vi "EMI_project_v3.vi"() -> ()   [LabVIEW 2020]
uses:
  <vilib>/Instr/_visa.llb/VISA Flush IO Buffer Mask.ctl
  <vilib>/Instr/_visa.llb/VISA Configure Serial Port (Instr).vi
panel:
  out "Fader 02 level":dbl
  out "Fader 01 level":dbl
  out "Gain Knob 02 level":dbl
  out "Gain knob 01 level":dbl
  out "manual mode led":bool
  out "Sound Balance Mode":bool
  in  "Gain Knob 02":dbl(knob) scale=0.0..270.0
  in  "Gain Knob 01":dbl(knob) scale=0.0..270.0
  in  "Fader 02 Slider":dbl(slide) scale=0.0..10.0
  in  "Fader 01 Slider":dbl(slide) scale=0.0..10.0
  out "Fader 02 Max":dbl
  out "Fader 01 Max":dbl
  in  "Calibrate":bool
  in  "stop":bool
  in  "VISA Resource":refnum<visa-resource-name>
  in  "?":bool
  in  "Gain 02":bool
  in  "?":bool
  in  "Gain 01":bool
  in  "?":bool
  in  "Fader 02":bool
  in  "?":bool
  in  "Fader 01":bool
  # "Automation System For Analog Audio Mixers"
  # "Calibration \nMode"
  # "Manual Mode"
  # "Sound Balance Mode"
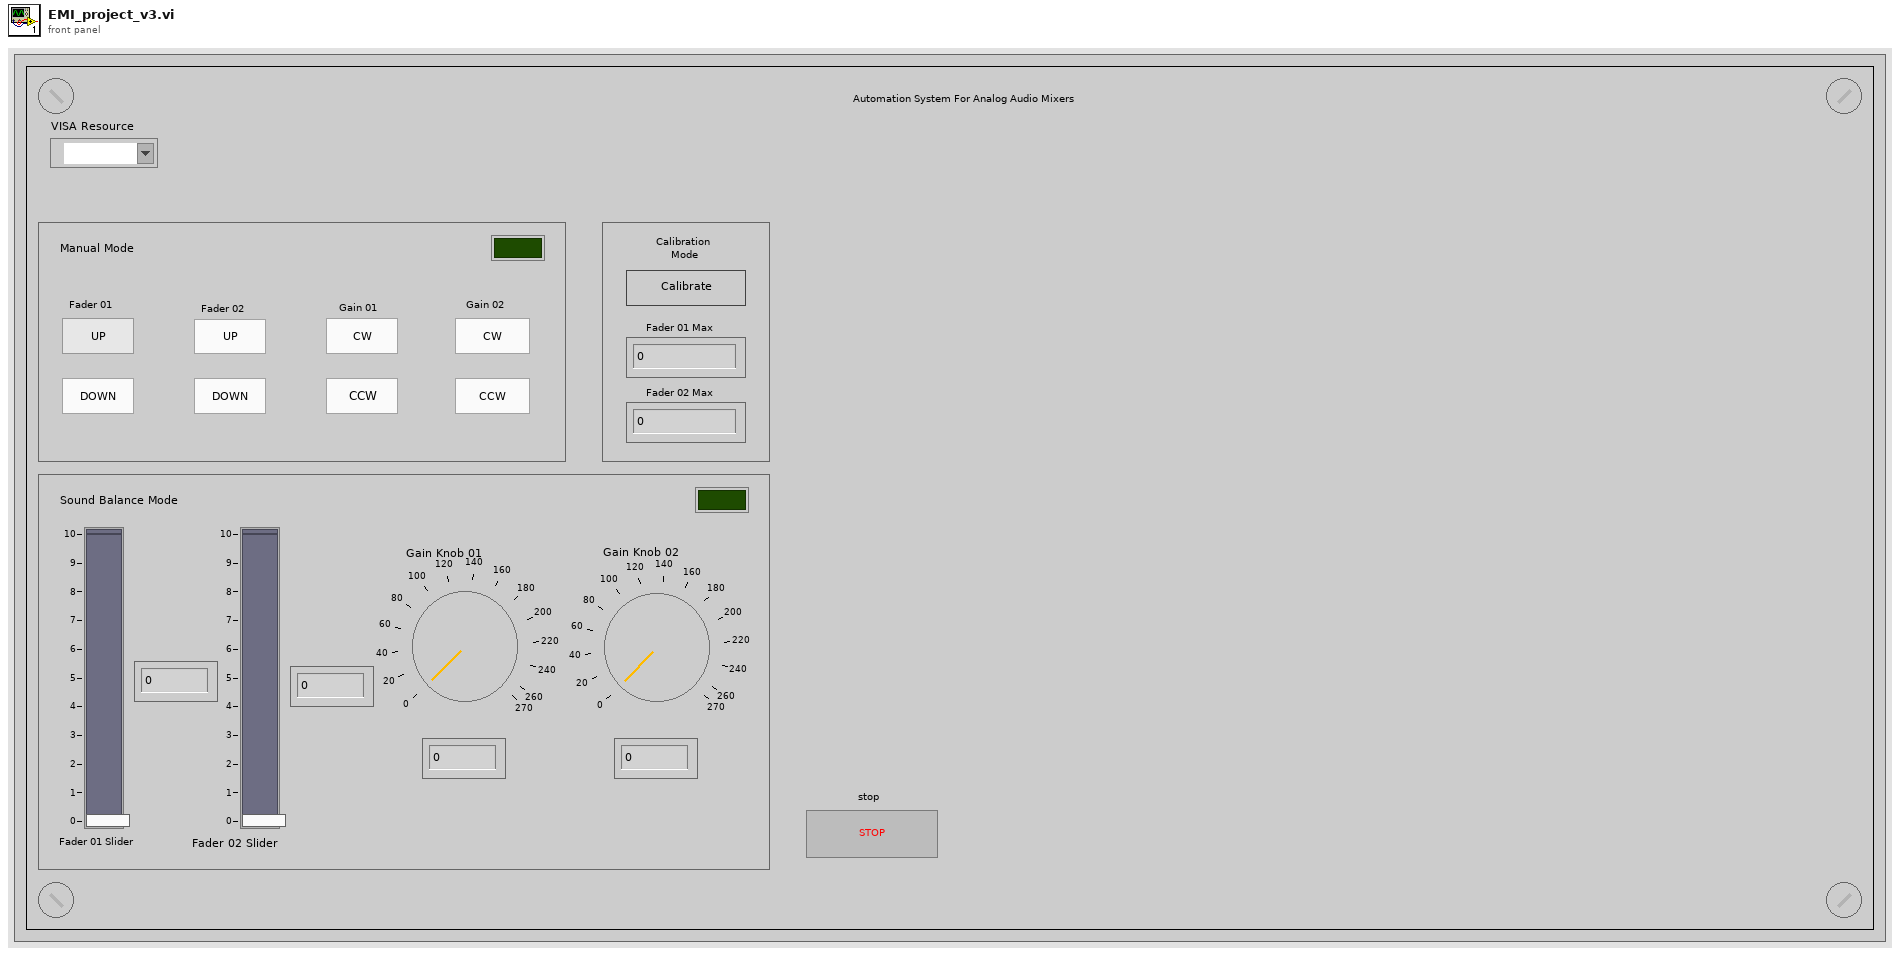
[diagram p1: front panel]
types:
  T1 = typedef "VISA Flush IO Buffer Mask.ctl" = u16
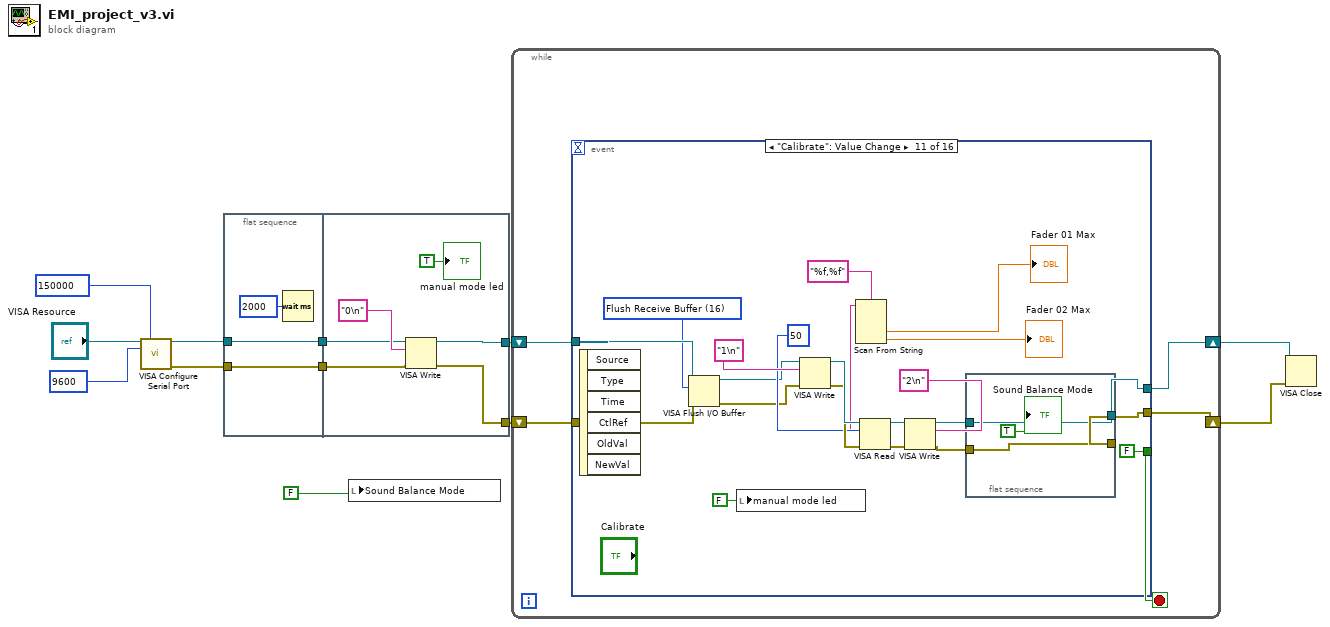
[diagram p0: block diagram]
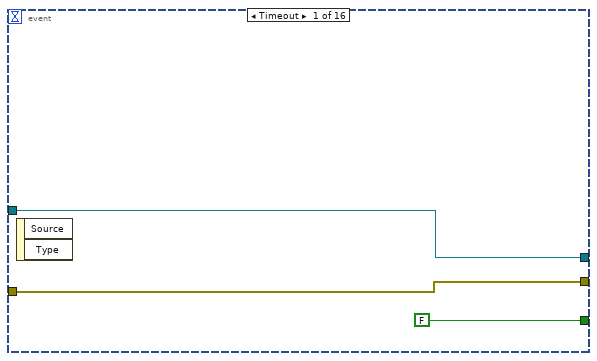
[diagram p2: hidden frame]
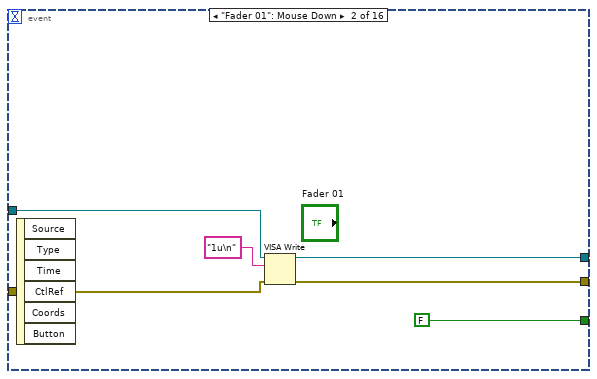
[diagram p3: hidden frame]
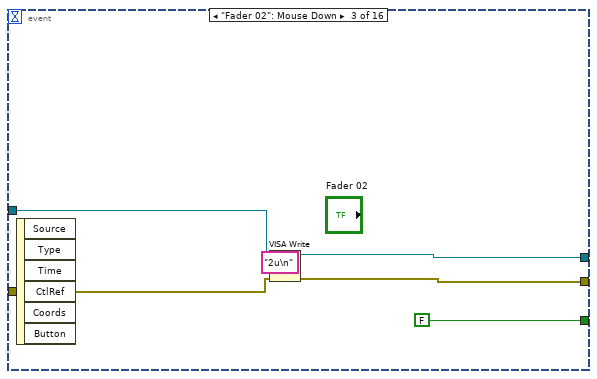
[diagram p4: hidden frame]
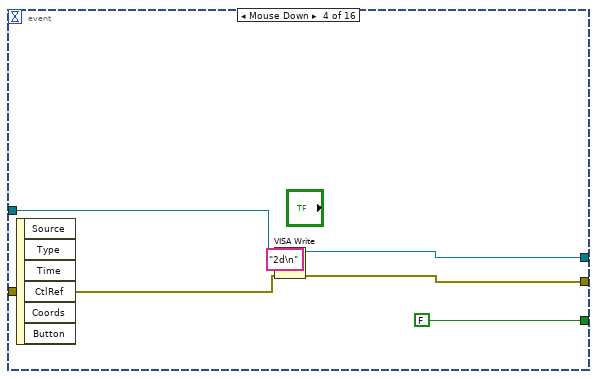
[diagram p5: hidden frame]
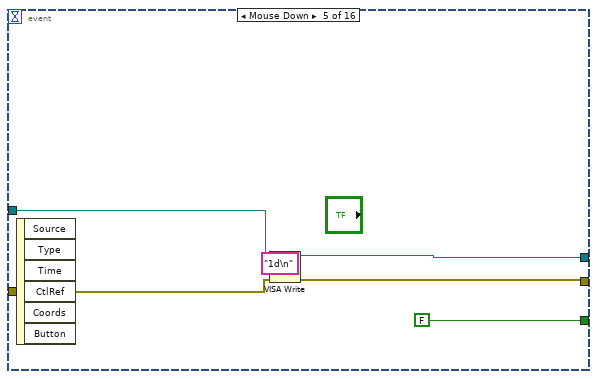
[diagram p6: hidden frame]
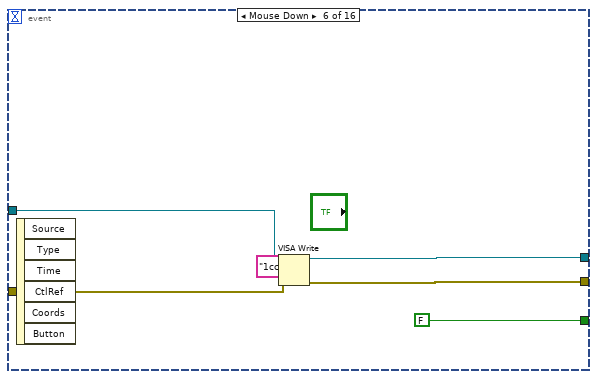
[diagram p7: hidden frame]
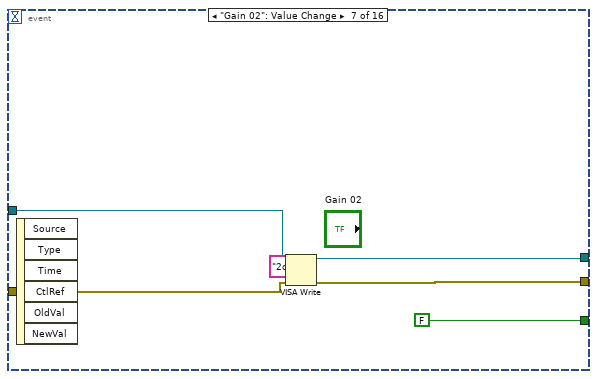
[diagram p8: hidden frame]
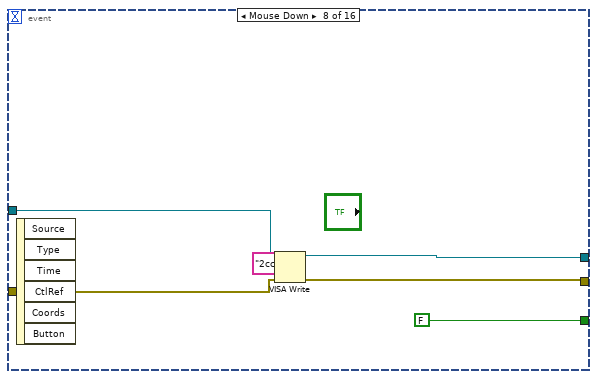
[diagram p9: hidden frame]
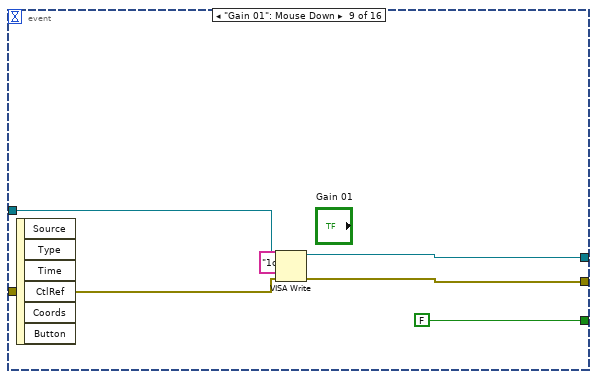
[diagram p10: hidden frame]
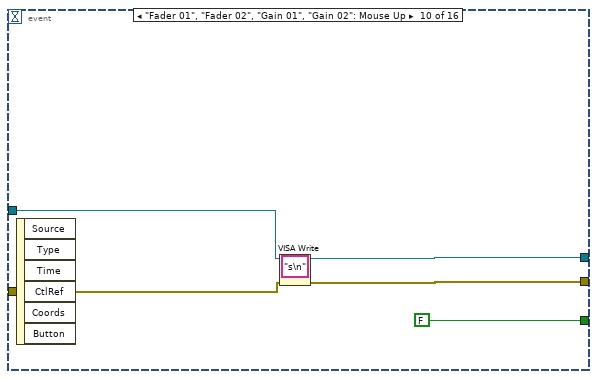
[diagram p11: hidden frame]
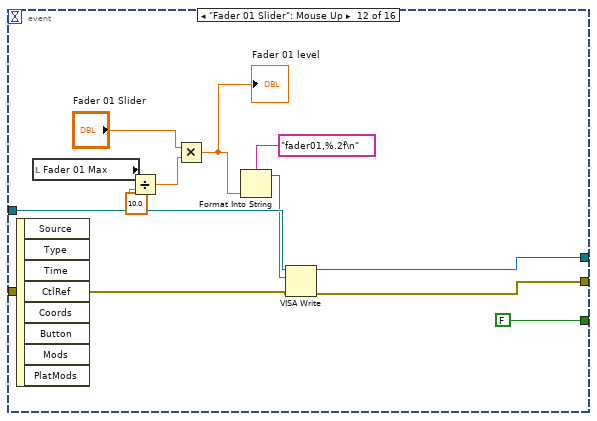
[diagram p12: hidden frame]
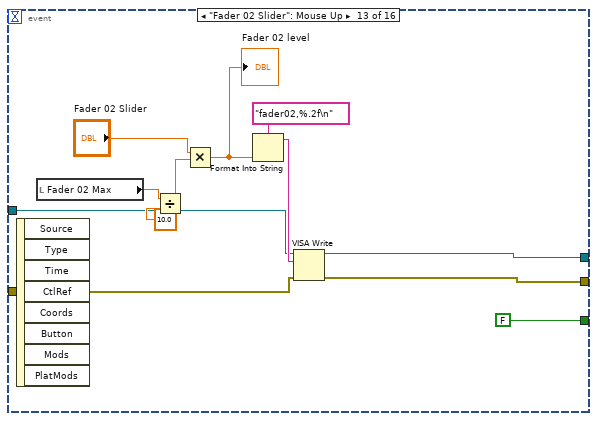
[diagram p13: hidden frame]
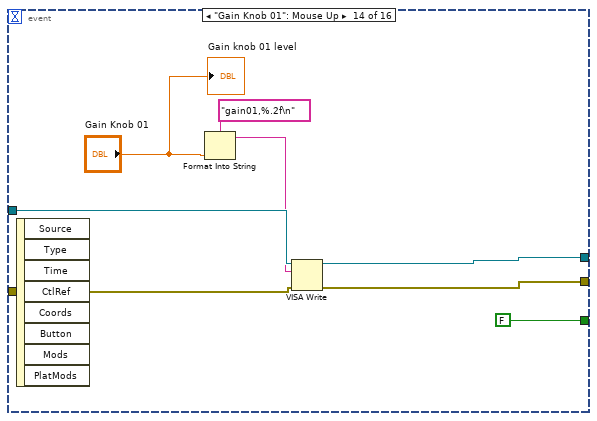
[diagram p14: hidden frame]
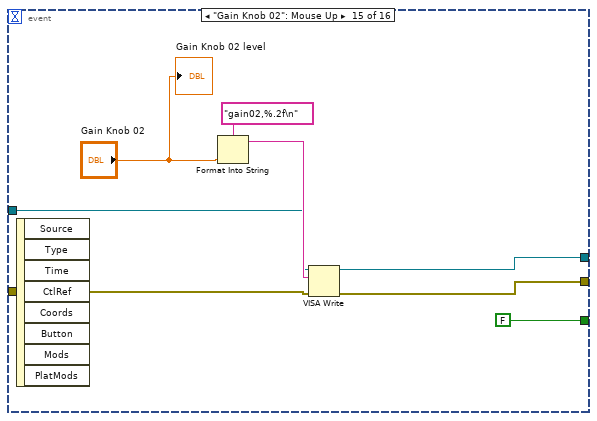
[diagram p15: hidden frame]
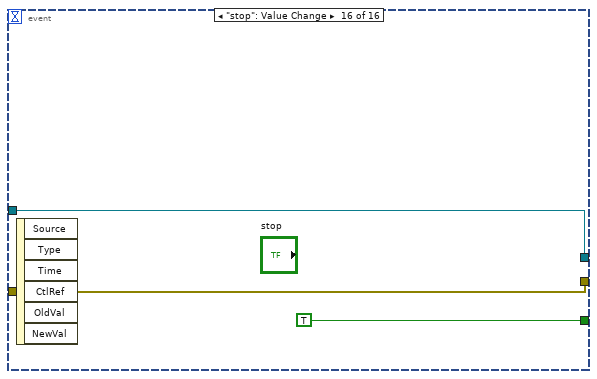
[diagram p16: hidden frame]
diagram:
  n1 = call-poly "VISA Configure Serial Port"("VISA resource name"="VISA Resource", "timeout (10sec)"=u32 150000, "baud rate (9600)"=u32 9600) -> ("VISA resource name out"=w6:refnum<visa-resource-name>, "error out"=w5:errorcluster)  [unwired: 11 in]
  n2 = flat-sequence {
    tunnel: w5 -> [w14]
    tunnel: w6 -> [w15]
    tunnel: [w15] -> w4
    tunnel: [w14] -> w3
    tunnel: [w20] -> w10
    tunnel: [w19] -> w9
    tunnel: w4 -> [w18]
    tunnel: w3 -> [w17]
    frame #0 {
      n3 = Wait (ms)(milliseconds to wait=u32 2000) -> ()  [unwired: 1 out]
    }
    frame #1 {
      n4 = VISA Write(VISA resource name=w18, write buffer="0\n", error in (no error)=w17) -> (VISA resource name out=w20:refnum<visa-resource-name>, error out=w19:errorcluster)  [unwired: 1 out]
      "manual mode led" <- TRUE
    }
  }
  n5 = local write "Sound Balance Mode"(FALSE) -> ()
  n6 = while {
    shift-right: [w24] -> w8
    shift-left: w10 -> [w26]
    shift-right: [w23] -> w7
    shift-left: w9 -> [w25]
    stop <- w22 stop-if-true
    n7 = event shown="[10] \"Calibrate\": Value Change" {
      selector: _ -> [_ _ _ _ _ _ _ _ _ _ _ _ _ _ _ _]
      dyn-events: _ -> [_ _ _ _ _ _ _ _ _ _ _ _ _ _ _ _]
      timeout: _ -> [_ _ _ _ _ _ _ _ _ _ _ _ _ _ _ _]
      tunnel: w26 -> [w29 w35 w39 w45 w53 w56 w63 w69 w75 w81 w97 w115 w126 w139 w146 w150]
      tunnel: w25 -> [w28 w34 w38 w44 w52 w57 w62 w68 w74 w80 w96 w114 w125 w138 w145 w149]
      tunnel: [w29 w32 w41 w47 w50 w59 w65 w71 w77 w83 w88 w111 w123 w136 w143 w150] -> w24
      tunnel: [w28 w31 w40 w46 w51 w58 w64 w70 w76 w82 w85 w113 w124 w137 w144 w149] -> w23
      tunnel: [FALSE FALSE FALSE FALSE FALSE FALSE FALSE FALSE FALSE FALSE FALSE FALSE FALSE FALSE FALSE TRUE] -> w22
      event Timeout {
        n8 = event-data() -> ()  [unwired: 1 in, 2 out]
      }
      event "Fader 01": Mouse Down {
        n9 = event-data() -> ()  [unwired: 1 in, 6 out]
        n10 = VISA Write(VISA resource name=w35, write buffer="1u\n", error in (no error)=w34) -> (VISA resource name out=w32:refnum<visa-resource-name>, error out=w31:errorcluster)  [unwired: 1 out]
      }
      event "Fader 02": Mouse Down {
        n11 = event-data() -> ()  [unwired: 1 in, 6 out]
        n12 = VISA Write(VISA resource name=w39, write buffer="2u\n", error in (no error)=w38) -> (VISA resource name out=w41:refnum<visa-resource-name>, error out=w40:errorcluster)  [unwired: 1 out]
      }
      event Mouse Down {
        n13 = event-data() -> ()  [unwired: 1 in, 6 out]
        n14 = VISA Write(VISA resource name=w45, write buffer="2d\n", error in (no error)=w44) -> (VISA resource name out=w47:refnum<visa-resource-name>, error out=w46:errorcluster)  [unwired: 1 out]
      }
      event Mouse Down {
        n15 = event-data() -> ()  [unwired: 1 in, 6 out]
        n16 = VISA Write(VISA resource name=w53, write buffer="1d\n", error in (no error)=w52) -> (VISA resource name out=w50:refnum<visa-resource-name>, error out=w51:errorcluster)  [unwired: 1 out]
      }
      event Mouse Down {
        n17 = event-data() -> ()  [unwired: 1 in, 6 out]
        n18 = VISA Write(VISA resource name=w56, write buffer="1ccw\n", error in (no error)=w57) -> (VISA resource name out=w59:refnum<visa-resource-name>, error out=w58:errorcluster)  [unwired: 1 out]
      }
      event "Gain 02": Value Change {
        n19 = event-data() -> ()  [unwired: 1 in, 6 out]
        n20 = VISA Write(VISA resource name=w63, write buffer="2cw\n", error in (no error)=w62) -> (VISA resource name out=w65:refnum<visa-resource-name>, error out=w64:errorcluster)  [unwired: 1 out]
      }
      event Mouse Down {
        n21 = event-data() -> ()  [unwired: 1 in, 6 out]
        n22 = VISA Write(VISA resource name=w69, write buffer="2ccw\n", error in (no error)=w68) -> (VISA resource name out=w71:refnum<visa-resource-name>, error out=w70:errorcluster)  [unwired: 1 out]
      }
      event "Gain 01": Mouse Down {
        n23 = event-data() -> ()  [unwired: 1 in, 6 out]
        n24 = VISA Write(VISA resource name=w75, write buffer="1cw\n", error in (no error)=w74) -> (VISA resource name out=w77:refnum<visa-resource-name>, error out=w76:errorcluster)  [unwired: 1 out]
      }
      event "Fader 01", "Fader 02", "Gain 01", "Gain 02": Mouse Up {
        n25 = event-data() -> ()  [unwired: 1 in, 6 out]
        n26 = VISA Write(VISA resource name=w81, write buffer="s\n", error in (no error)=w80) -> (VISA resource name out=w83:refnum<visa-resource-name>, error out=w82:errorcluster)  [unwired: 1 out]
      }
      event "Calibrate": Value Change {
        w93 = T1 16 items=["Flush Receive Buffer"=16, "Write Transmit Buffer to Device"=32, "Flush Receive Buffer (No I/O)"=64, "Flush Transmit Buffer"=128] ("Mask")
        n27 = event-data() -> ()  [unwired: 1 in, 6 out]
        n28 = VISA Flush I/O Buffer(VISA resource name=w97, mask (16)=w93, error in (no error)=w96) -> (VISA resource name out=w95:refnum<visa-resource-name>, error out=w94:errorcluster)
        n29 = local write "manual mode led"(FALSE ("manual mode led")) -> ()
        n30 = VISA Write(VISA resource name=w95, write buffer="1\n", error in (no error)=w94) -> (VISA resource name out=w104:refnum<visa-resource-name>, error out=w103:errorcluster)  [unwired: 1 out]
        n31 = VISA Read(VISA resource name=w104, byte count=u32 50, error in (no error)=w103) -> (VISA resource name out=w92:refnum<visa-resource-name>, read buffer=w101:string, error out=w91:errorcluster)  [unwired: 1 out]
        n32 = Scan From String(format string="%f,%f", input string=w101) -> (output 1=→"Fader 01 Max":dbl, output 2=→"Fader 02 Max":dbl)  [unwired: 4 in, 3 out]
        n33 = VISA Write(VISA resource name=w92, write buffer="2\n", error in (no error)=w91) -> (VISA resource name out=w87:refnum<visa-resource-name>, error out=w86:errorcluster)  [unwired: 1 out]
        n34 = flat-sequence {
          tunnel: [w107] -> w88
          tunnel: w87 -> [w107]
          tunnel: w86 -> [w106]
          tunnel: [w106] -> w85
          frame #0 {
            "Sound Balance Mode" <- TRUE
          }
        }
      }
      event "Fader 01 Slider": Mouse Up {
        n35 = event-data() -> ()  [unwired: 1 in, 8 out]
        n36 = local read "Fader 01 Max"() -> (w119:dbl)
        n37 = Divide(x=w119, y=10.0) -> (x/y=w116:dbl)
        n38 = Multiply(x="Fader 01 Slider", y=w116) -> (x*y=w109:dbl)
        "Fader 01 level" <- w109
        n39 = Format Into String(format string="fader01,%.2f\n", w109) -> (resulting string=w110:string)  [unwired: 2 in, 1 out]
        n40 = VISA Write(VISA resource name=w115, write buffer=w110, error in (no error)=w114) -> (VISA resource name out=w111:refnum<visa-resource-name>, error out=w113:errorcluster)  [unwired: 1 out]
      }
      event "Fader 02 Slider": Mouse Up {
        n41 = event-data() -> ()  [unwired: 1 in, 8 out]
        n42 = local read "Fader 02 Max"() -> (w132:dbl)
        n43 = Divide(x=w132, y=10.0) -> (x/y=w129:dbl)
        n44 = Multiply(x="Fader 02 Slider", y=w129) -> (x*y=w121:dbl)
        "Fader 02 level" <- w121
        n45 = Format Into String(format string="fader02,%.2f\n", w121) -> (resulting string=w127:string)  [unwired: 2 in, 1 out]
        n46 = VISA Write(VISA resource name=w126, write buffer=w127, error in (no error)=w125) -> (VISA resource name out=w123:refnum<visa-resource-name>, error out=w124:errorcluster)  [unwired: 1 out]
      }
      event "Gain Knob 01": Mouse Up {
        n47 = event-data() -> ()  [unwired: 1 in, 8 out]
        n48 = Format Into String(format string="gain01,%.2f\n", "Gain Knob 01") -> (resulting string=w135:string)  [unwired: 2 in, 1 out]
        n49 = VISA Write(VISA resource name=w139, write buffer=w135, error in (no error)=w138) -> (VISA resource name out=w136:refnum<visa-resource-name>, error out=w137:errorcluster)  [unwired: 1 out]
        "Gain knob 01 level" <- "Gain Knob 01"
      }
      event "Gain Knob 02": Mouse Up {
        n50 = event-data() -> ()  [unwired: 1 in, 8 out]
        n51 = Format Into String(format string="gain02,%.2f\n", "Gain Knob 02") -> (resulting string=w147:string)  [unwired: 2 in, 1 out]
        n52 = VISA Write(VISA resource name=w146, write buffer=w147, error in (no error)=w145) -> (VISA resource name out=w143:refnum<visa-resource-name>, error out=w144:errorcluster)  [unwired: 1 out]
        "Gain Knob 02 level" <- "Gain Knob 02"
      }
      event "stop": Value Change {
        n53 = event-data() -> ()  [unwired: 1 in, 6 out]
      }
    }
  }
  n54 = VISA Close(VISA resource name=w8, error in (no error)=w7) -> ()  [unwired: 1 out]
